vi "NVH Inputs Controls Buffer.vi"(8 "Error in":string[][](array[string]), 9 "NVH Inputs":bool[](array[boolean]), 10 "NVHK Inputs Control":T2[](array[typedef]), 11 "Mode":T1) -> (0 "Error out":string[][](array[string]), 2 "NVH Single Input":bool, 3 "NVH Inputs Out":bool[](array[boolean]))   [LabVIEW 2018]
uses:
  02.Type Def's/NVH Digital Input.ctl
  02.Type Def's/NVH Mode Control.ctl
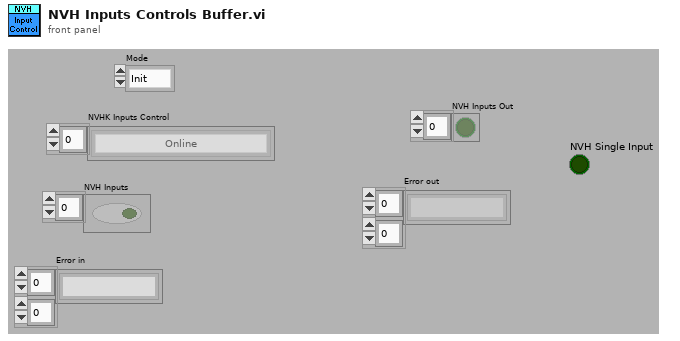
[diagram p1: front panel]
types:
  T1 = typedef "NVH Mode Control.ctl" = enum16{"Init", "Write", "Write String", "Read"}
  T2 = typedef "NVH Digital Input.ctl" = enum16{"Online", "Pass", "Fail", "Testing", "Ready for Model", "Error Bit 1", "Error Bit 2", "Error Bit 3", "Failure Bit 1", "Failure Bit 2", "Failure Bit 3", "Failure Bit 4", "Echo Bit 1", "Echo Bit 2", "Echo Bit 3", "Echo Bit 4", "Serial Number Read Ok", "Ready for Serrial Number"}
  T3 = cluster{"B&K Inputs":bool[], "Error Message":string[][]}
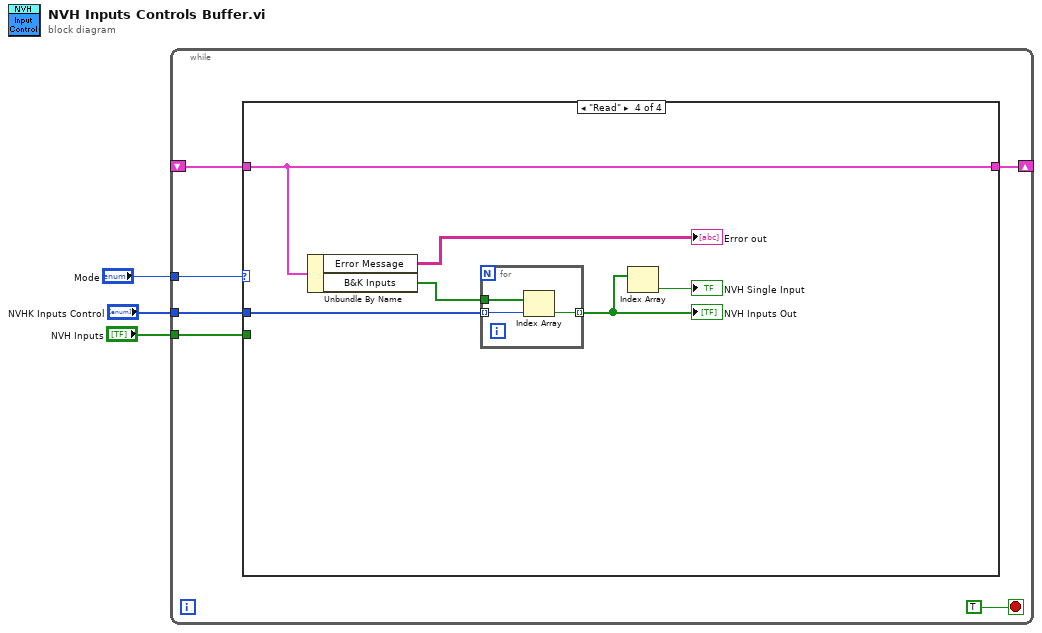
[diagram p0: block diagram]
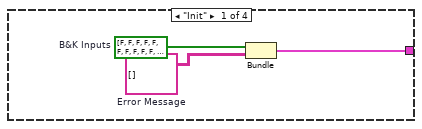
[diagram p2: hidden frame]
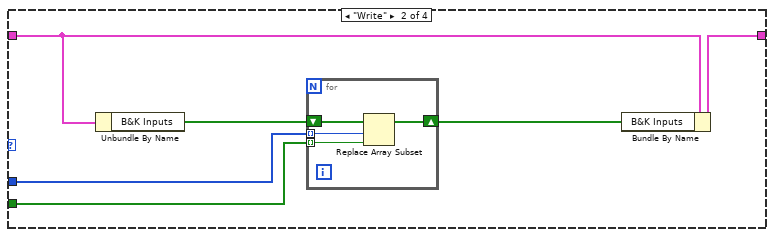
[diagram p3: hidden frame]
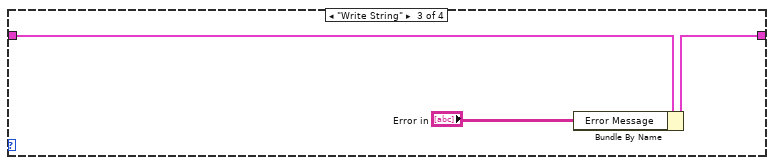
[diagram p4: hidden frame]
diagram:
  n1 = while {
    tunnel: "Mode" -> [w8]
    shift-right: [w6] -> _
    shift-left: _ -> [w7]
    tunnel: "NVHK Inputs Control" -> [w5]
    tunnel: "NVH Inputs" -> [w4]
    stop <- TRUE stop-if-true
    n2 = case shown="\"Read\"" w8 {
      tunnel: w7 -> [_ w15 w25 w31]
      tunnel: [w11 w14 w24 w31] -> w6
      tunnel: w5 -> [_ w17 _ w28]
      tunnel: w4 -> [_ w16 _ _]
      frame "Init" {
        w10 = string[][] []  # Error Message
        w12 = bool[] [FALSE, FALSE, FALSE, FALSE, FALSE, FALSE, FALSE, FALSE, FALSE, FALSE, FALSE, FALSE, FALSE, FALSE, FALSE, FALSE, FALSE, FALSE]  # B&K Inputs
        n3 = Bundle("B&K Inputs"=w12, "Error Message"=w10) -> (w11:T3)  [unwired: 1 out]
      }
      frame "Write" {
        n4 = Unbundle By Name(w15) -> ("B&K Inputs"=w18:bool[])
        n5 = for {
          shift-right: [w19] -> w13
          shift-left: w18 -> [w22]
          tunnel: w17 -> [w21] mode=indexing
          tunnel: w16 -> [w20] mode=indexing
          n6 = Replace Array Subset(array=w22, new element=w20, index=w21) -> (w19:bool[])
        }
        n7 = Bundle By Name(cluster=w15, "B&K Inputs"=w13) -> (w14:T3)
      }
      frame "Write String" {
        n8 = Bundle By Name(cluster=w25, "Error Message"="Error in") -> (w24:T3)
      }
      frame "Read" {
        n9 = Unbundle By Name(w31) -> ("Error Message"=→"Error out":string[][], "B&K Inputs"=w27:bool[])
        n10 = for {
          tunnel: w28 -> [w33] mode=indexing
          tunnel: w27 -> [w34]
          tunnel: [w32] -> w26 mode=indexing
          n11 = Index Array(array=w34, index=w33) -> (element=w32:bool)
        }
        "NVH Inputs Out" <- w26
        n12 = Index Array(array=w26) -> (element=→"NVH Single Input":bool)  [unwired: 1 in]
      }
    }
  }
